vi "DropButtonTimer.vi"(10 "action":enum16{"Get", "Start"}(ring)=enum."Start") -> (1 "Time elapsed":bool)   [LabVIEW 2014]
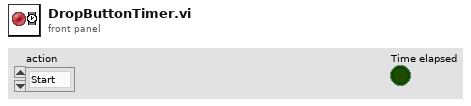
[diagram p1: front panel]
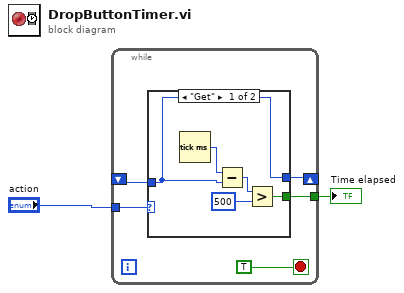
[diagram p0: block diagram]
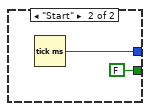
[diagram p2: hidden frame]
diagram:
  n1 = while {
    shift-right: [w5] -> _
    shift-left: _ -> [w4]
    tunnel: "action" -> [w6]
    tunnel: [w3] -> w1
    stop <- TRUE stop-if-true
    n2 = case shown="\"Get\"" w6 {
      tunnel: [w8 w14] -> w5
      tunnel: w4 -> [w8 _]
      tunnel: [w10 FALSE] -> w3
      frame "Get" {
        n3 = Tick Count (ms)() -> (millisecond timer value=w12:u32)
        n4 = Subtract(x=w12, y=w8) -> (x-y=w9:u32)
        n5 = Greater?(x=w9, y=u32 500) -> (0:w10:bool)
      }
      frame "Start" {
        n6 = Tick Count (ms)() -> (millisecond timer value=w14:u32)
      }
    }
  }
  "Time elapsed" <- w1
